vi "tracks.vi"(11 "project-param out 3":T1) -> (3 "delimited string":string)   [LabVIEW 2019]
uses:
  Project Parameters.ctl
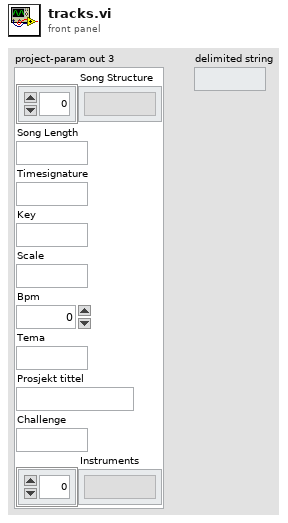
[diagram p1: front panel]
types:
  T1 = typedef "Project Parameters.ctl" = cluster{"Song Structure":string[], "Song Length":string, "Timesignature":string, "Key":string, "Scale":string, "Bpm":i32, "Tema":string, "Prosjekt tittel":string, "Challenge":string, "Instruments":string[]}
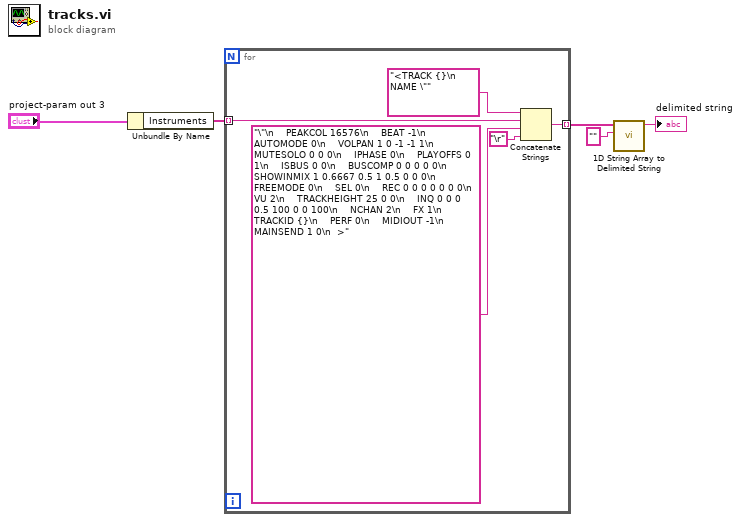
[diagram p0: block diagram]
diagram:
  n1 = Unbundle By Name("project-param out 3") -> ("Instruments"=w2:string[])
  n2 = for {
    tunnel: w2 -> [w9] mode=indexing
    tunnel: [w7] -> w4 mode=indexing
    n3 = Concatenate Strings("<TRACK {}\n    NAME \"", w9, "\"\n    PEAKCOL 16576\n    BEAT -1\n    AUTOMODE 0\n    VOLPAN 1 0 -1 -1 1\n    MUTESOLO 0 0 0\n    IPHASE 0\n    PLAYOFFS 0 1\n    ISBUS 0 0\n    BUSCOMP 0 0 0 0 0\n    SHOWINMIX 1 0.6667 0.5 1 0.5 0 0 0\n    FREEMODE 0\n    SEL 0\n    REC 0 0 0 0 0 0 0\n    VU 2\n    TRACKHEIGHT 25 0 0\n    INQ 0 0 0 0.5 100 0 0 100\n    NCHAN 2\n    FX 1\n    TRACKID {}\n    PERF 0\n    MIDIOUT -1\n    MAINSEND 1 0\n  >", "\r") -> (w7:string)
  }
  n4 = call <vilib>:"1D String Array to Delimited String.vi"("delimiter"="", "string array"=w4) -> ("delimited string"=→"delimited string":string)  [unwired: 9 in]
